vi "mag graphs to tmag.vi"(10 "graphs":T1) -> (2 "t-mag":cluster{dbl[], sgl[]})   [LabVIEW 2017]
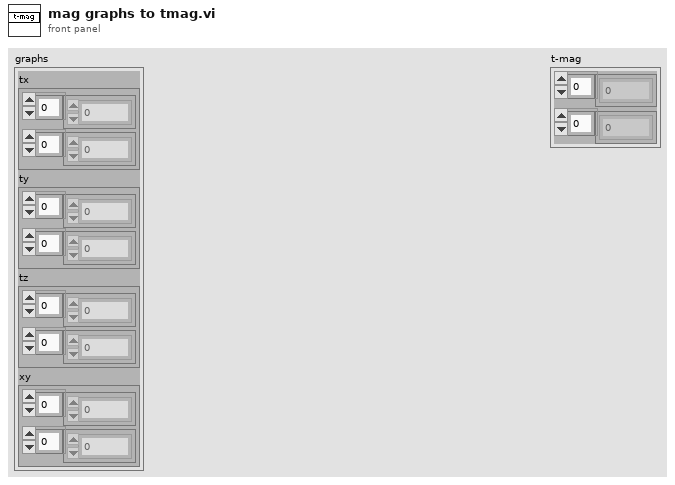
[diagram p1: front panel]
types:
  T1 = cluster{"tx":cluster{dbl[], sgl[]}, "ty":cluster{dbl[], sgl[]}, "tz":cluster{dbl[], sgl[]}, "xy":cluster{sgl[], sgl[]}}
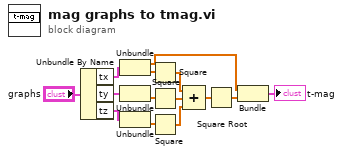
[diagram p0: block diagram]
diagram:
  n1 = Unbundle By Name("graphs") -> ("tx"=w13:cluster{dbl[], sgl[]}, "ty"=w12:cluster{dbl[], sgl[]}, "tz"=w11:cluster{dbl[], sgl[]})
  n2 = Unbundle(w13) -> (w3:dbl[], w10:sgl[])
  n3 = Unbundle(w12) -> (w9:sgl[])  [unwired: 1 out]
  n4 = Unbundle(w11) -> (w8:sgl[])  [unwired: 1 out]
  n5 = Square(x=w10) -> (x^2=w7:sgl[])
  n6 = Square(x=w9) -> (x^2=w6:sgl[])
  n7 = Square(x=w8) -> (x^2=w5:sgl[])
  n8 = Compound Arithmetic op=ADD(w7, w6, w5) -> (w4:sgl[])
  n9 = Square Root(x=w4) -> (sqrt(x)=w1:sgl[])
  n10 = Bundle(w3, w1) -> (→"t-mag":cluster{dbl[], sgl[]})  [unwired: 1 in]
